vi "Measurement UI.vi"() -> ()   [LabVIEW 2025, in "Automotive Vision UI.lvlib"]
uses:
  Automotive Vision UI.lvlib
  <vilib>/gRPC/LabVIEW gRPC Library/Shared/grpcId.ctl
  <vilib>/vision/Image Controls.llb/IMAQ Image.ctl
  auto vision config.ctl
  Automotive-Vision-OOBService_client/RPC Messages/hwval_BoolRequest.ctl
  Automotive-Vision-OOBService_client/RPC Messages/hwval_ExportRequest.ctl
  Automotive-Vision-OOBService_client/RPC Messages/hwval_ExportTypeRequest.ctl
  Automotive-Vision-OOBService_client/RPC Messages/hwval_ExportFileType.ctl
  <vilib>/gRPC/LabVIEW gRPC Library/grpc-lvsupport-release.lvlib
  Automotive-Vision-OOBService_client/Automotive-Vision-OOBService_client.lvlib
panel:
  in  "REGISTERS":string[][](table)
  in  "FRAME COUNT BYTES":u32[](array[numeric]) format="%02x"
  in  "config":string
  out "WIDTH":u64
  out "HEIGHT":u64
  out "Numeric":i32
  out "error out":errorcluster
  in  "GRPC status":string
  out "OOB gRPC Port":i32
  in  "BITFILE":string="IMAGE RESOLUTION: 800x600 - RAW12"
  out "Available SI Devices":string[][](array[string])
  in  "RIO HANDLER":string
  out "BYTES ACQUIRED":u64 format="%#.6p"
  out "ERROR":bool
  out "IMAGE PIXEL DATA":u32[](array[numeric])
  in  "IMAGE SAVE FORMAT":u32(ring) items=["PNG", "RAW LLP"]
  out "FRAME COUNT":u64
  out "IMAGE DATA":string
  in  "PAUSE":bool
  in  "CAPTURE":bool
  in  "PATH TO IMAGE CAPTURE":path
  in  "SERIAL CHANNEL":string="SI1"
  out "SOURCE RATE (fps)":dbl
  out "STATE MESSAGE":string
  out "POC CURRENT (A)":dbl
  out "POC VOLTAGE (V)":dbl
  out "ACQ. DURATION (s)":dbl
  out "ACQ. IN PROGRESS":bool
  out "DISPLAY":T1(plugin-control)
  # "CONFIGURATION"
  # "Image path parameters"
  # "CONTROL"
  # "MONITOR"
  # "STATUS"
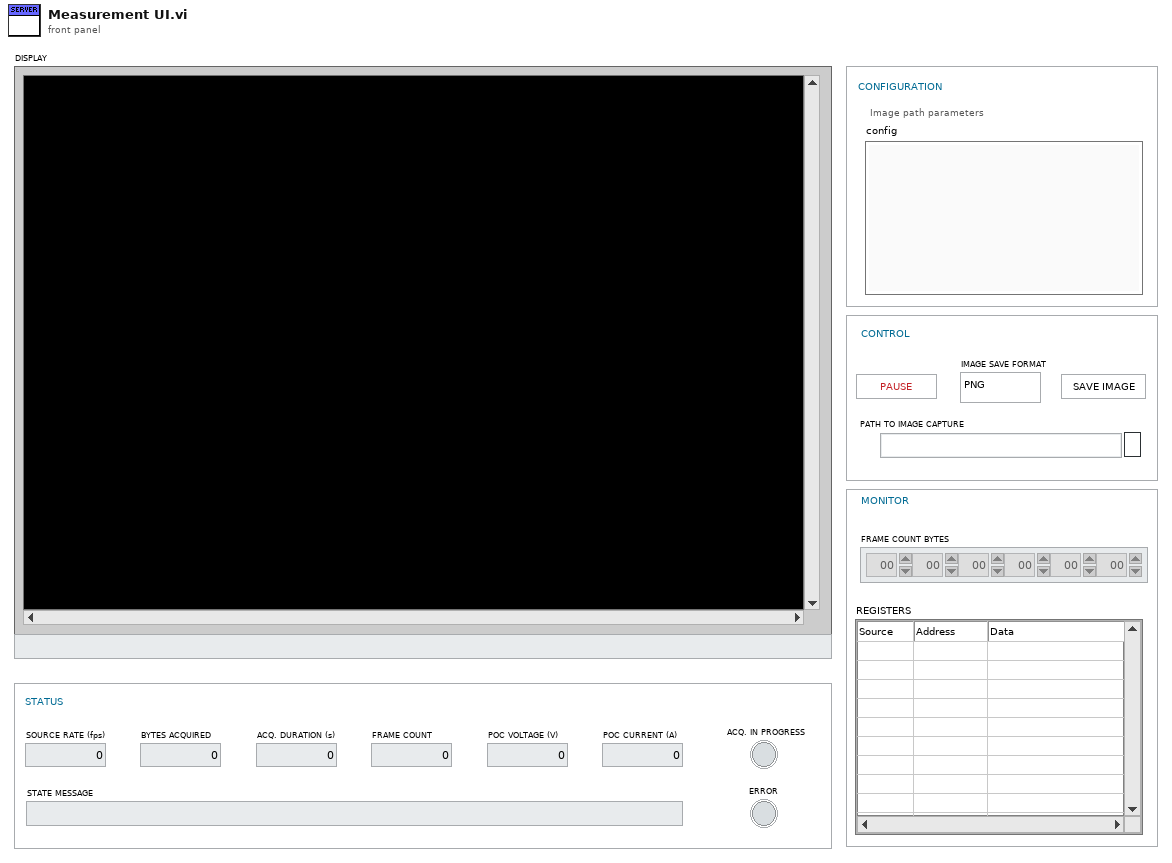
[diagram p1: front panel]
types:
  T1 = typedef "IMAQ Image.ctl" = refnum<image>
  T2 = typedef "Automotive Vision UI.lvlib/auto vision config.ctl" = cluster{"RIO Device":string, "Serial Channel":string, "SERDES Script":string, "POC Source":u32, "CSI-2 Data Source":u32, "Lane Count":u32, "Reference Clock":dbl, "Image Data Type":u32, "Interpretation":u32, "Pattern":u32, "Algorithm":u32, "Virtual Channel":u32, "Embedded Data":cluster{"Pre-embedded Lines":dbl, "Pre-embedded Line Length":dbl, "Post-embedded Lines":dbl, "Post-embedded Line Length":dbl, "Frame Count":cluster{"Line":dbl, "Offset":dbl, "Byte Count":dbl}}}
  T3 = typedef "grpc-lvsupport-release.lvlib/grpcId.ctl" = u64
  T4 = cluster{"pattern":i32, "algorithm":i32, "red gain":dbl, "green gain":dbl, "blue gain":dbl}
  T5 = typedef "Automotive-Vision-OOBService_client.lvlib/hwval_BoolRequest.ctl" = cluster{"BooleanData":bool}
  T6 = typedef "Automotive-Vision-OOBService_client.lvlib/hwval_ExportRequest.ctl" = cluster{"FilePath":string}
  T7 = typedef "Automotive-Vision-OOBService_client.lvlib/hwval_ExportTypeRequest.ctl" = cluster{"FileType":T8}
  T8 = typedef "Automotive-Vision-OOBService_client.lvlib/hwval_ExportFileType.ctl" = enum32{"EXPORT_PNG", "EXPORT_RAW"}
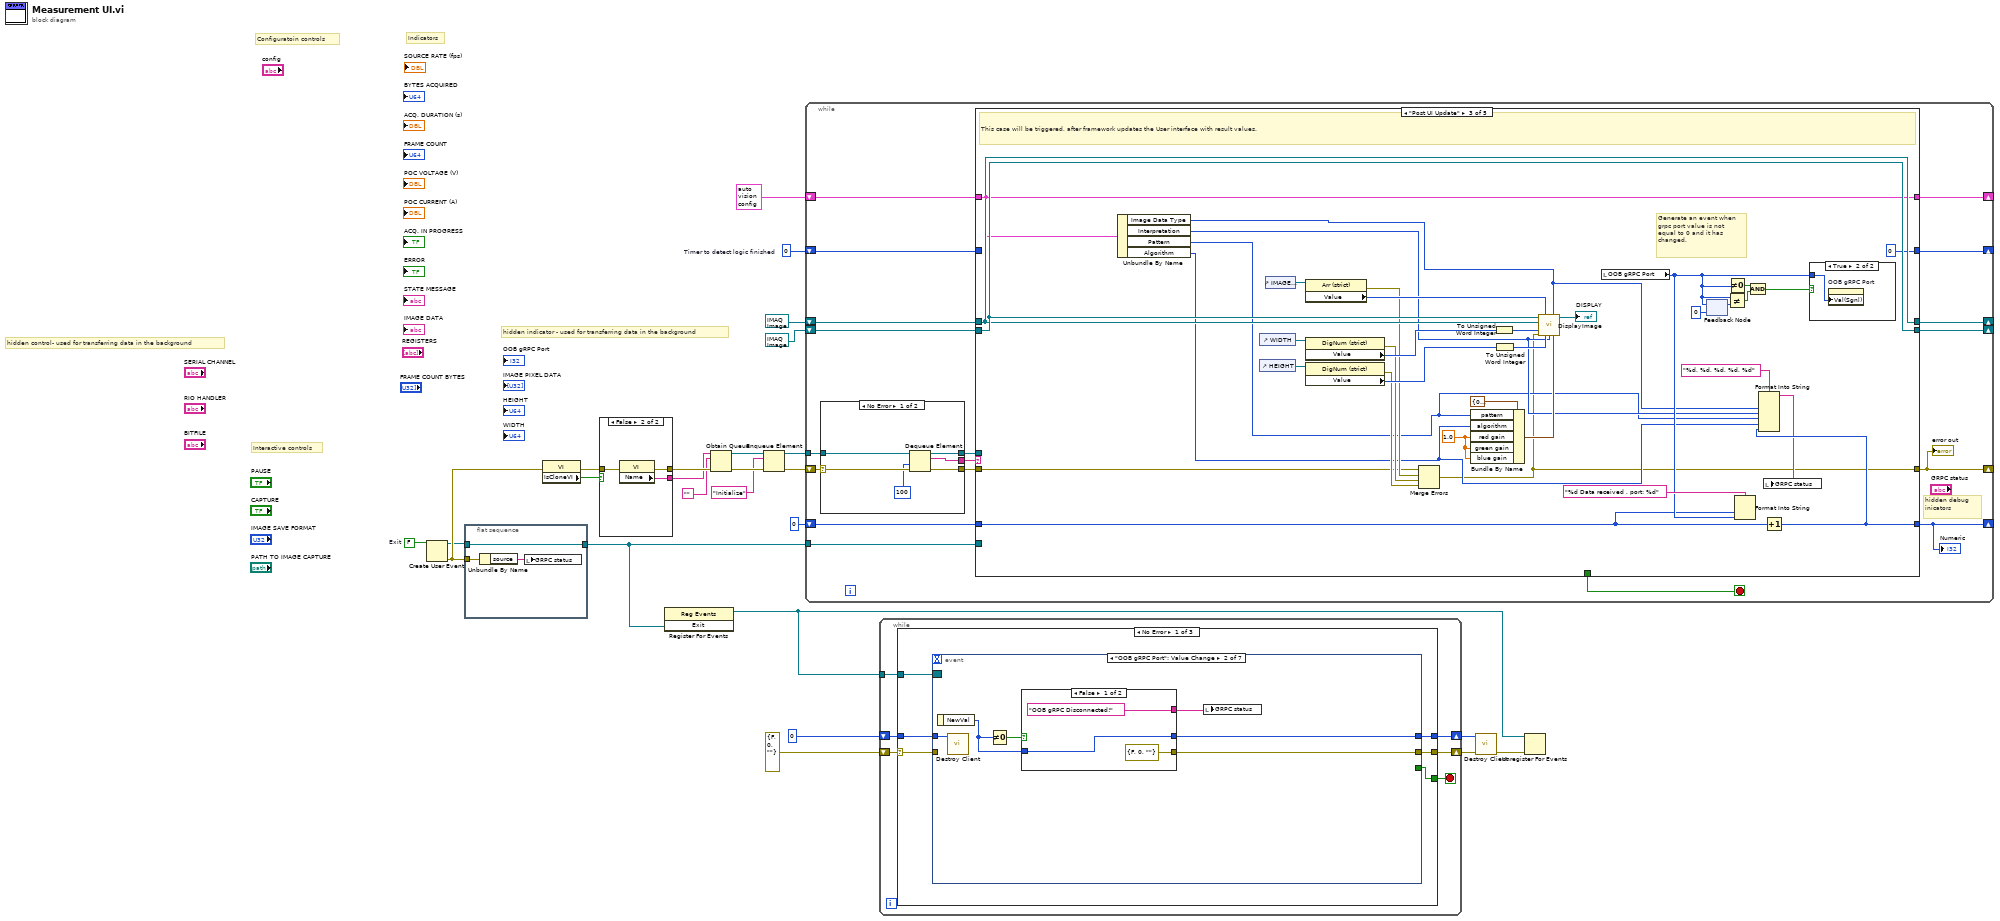
[diagram p0: block diagram]
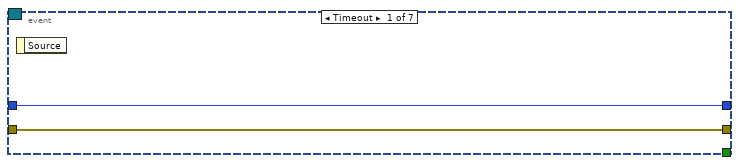
[diagram p2: hidden frame]
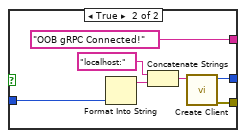
[diagram p3: hidden frame]
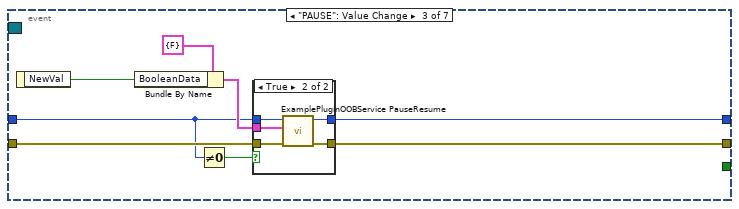
[diagram p4: hidden frame]
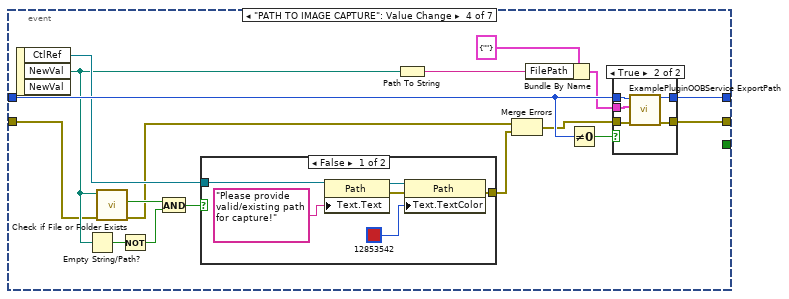
[diagram p6: hidden frame]
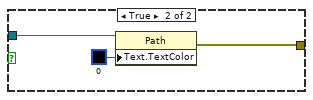
[diagram p7: hidden frame]
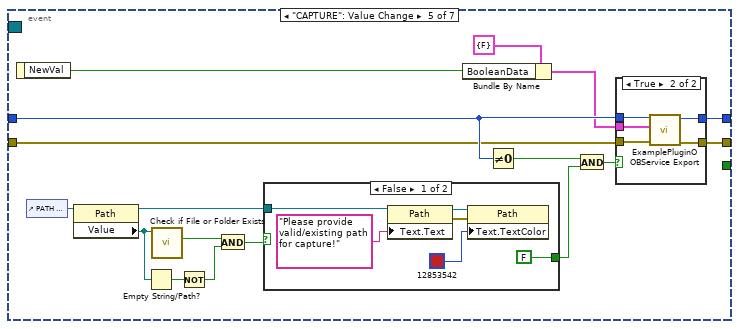
[diagram p9: hidden frame]
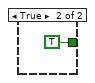
[diagram p10: hidden frame]
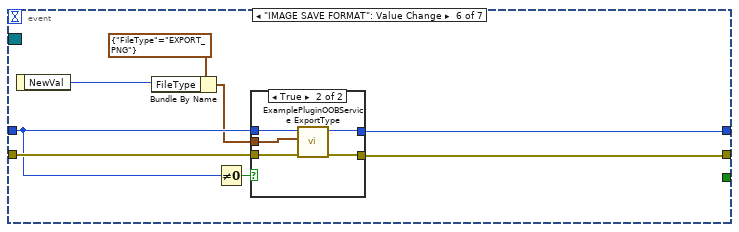
[diagram p12: hidden frame]
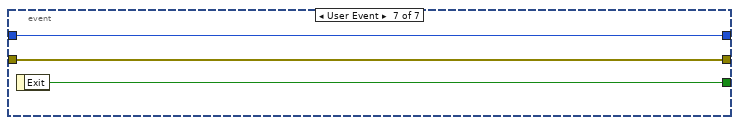
[diagram p14: hidden frame]
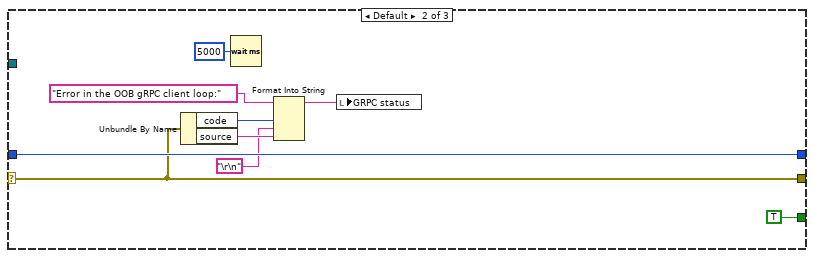
[diagram p15: hidden frame]
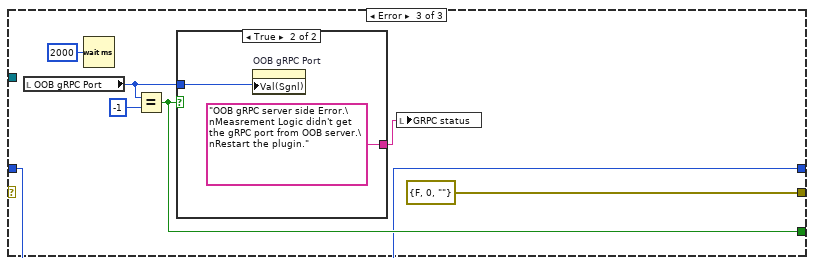
[diagram p16: hidden frame]
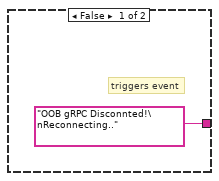
[diagram p17: hidden frame]
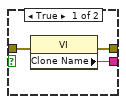
[diagram p18: hidden frame]
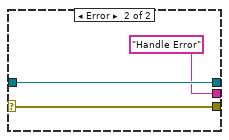
[diagram p19: hidden frame]
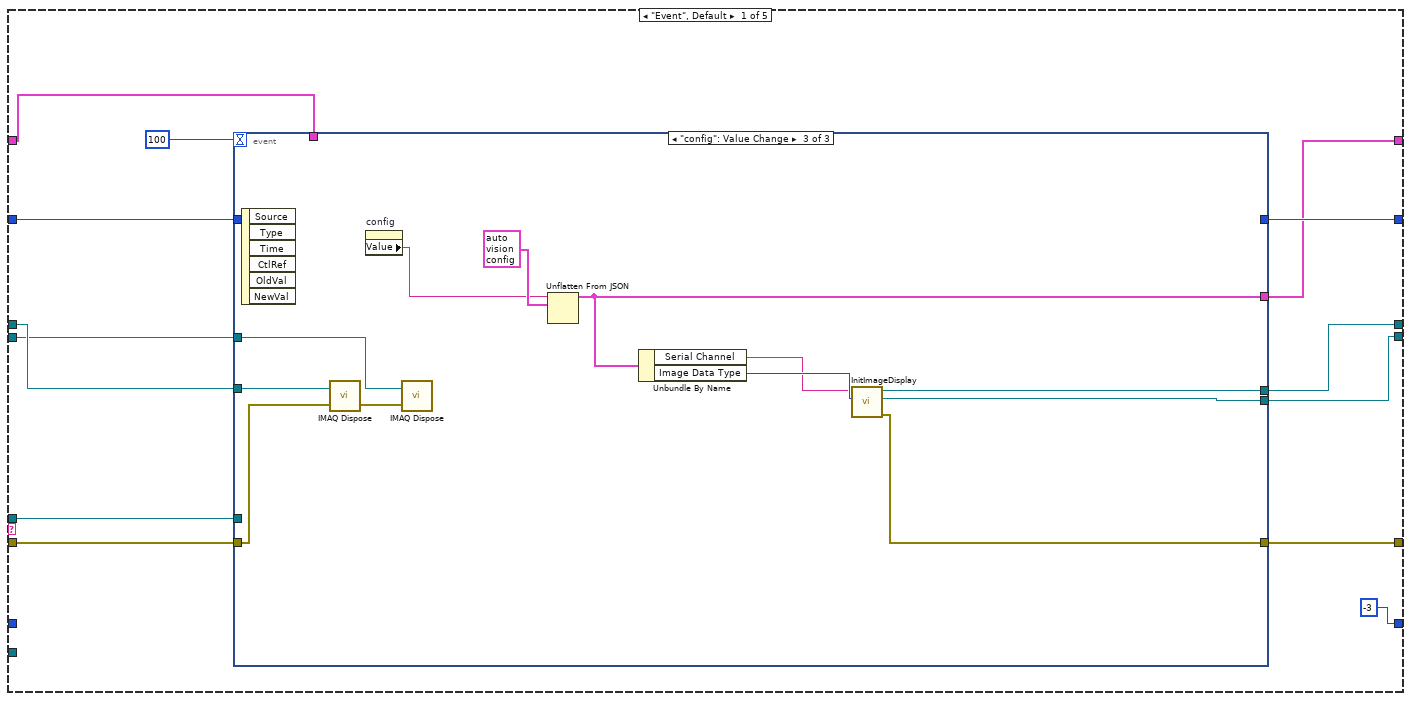
[diagram p20: hidden frame]
diagram:
  w6 = 0  # Timer to detect logic finished
  w15 = FALSE  # Exit
  # "Indicators"
  # "Configuratoin controls"
  # "Interactive controls"
  # "hidden indicator - used for transferring data in the background"
  # "hidden control- used for transferring data in the background"
  n1 = Create User Event(user event datatype=w15) -> (user event=w2:refnum<user-event>, error out=w8:errorcluster)  [unwired: 1 in]
  n2 = flat-sequence {
    tunnel: [w28] -> w9
    tunnel: w2 -> [w28]
    tunnel: w8 -> [w27]
    frame #0 {
      n3 = Unbundle By Name(w27) -> ("source"=w26:string)
      n4 = local write "GRPC status"(w26) -> ()
    }
  }
  n5 = property on="Property Node" class="VI"(error in=w8) -> (error out=w16:errorcluster, "IsCloneVI"=w17:bool)  [unwired: 1 in, 1 out]
  n6 = case shown="False" w17 {
    tunnel: [w31 w34] -> w25
    tunnel: [w30 w33] -> w24
    tunnel: w16 -> [w29 w32]
    frame True {
      n7 = property on="Property Node" class="VI"(error in=w29) -> (error out=w31:errorcluster, "Clone Name"=w30:string)  [unwired: 1 in, 1 out]
    }
    frame False {
      n8 = property on="Property Node" class="VI"(error in=w32) -> (error out=w34:errorcluster, "Name"=w33:string)  [unwired: 1 in, 1 out]
    }
  }
  n9 = register-events(w9) -> (reference out=w14:refnum<event-registration>)  [unwired: 2 in, 1 out]
  n10 = Obtain Queue(name (unnamed)=w24, element data type="" ("Empty String Constant"), error in (no error)=w25) -> (queue out=w21:refnum<queue>, error out=w23:errorcluster)  [unwired: 2 in, 1 out]
  n11 = Enqueue Element(queue=w21, element="Initialize", error in (no error)=w23) -> (queue out=w20:refnum<queue>, error out=w22:errorcluster)  [unwired: 1 in, 1 out]
  n12 = while {
    shift-right: [w41] -> _
    shift-left: w22 -> [w52]
    tunnel: w20 -> [w50]
    shift-right: [w43] -> _
    shift-left: T1 refnum ("Image Out Grayscale") -> [w45]
    shift-right: [w46] -> _
    shift-left: T1 refnum ("Image Out Grayscale") -> [w44]
    tunnel: w9 -> [w42]
    shift-right: [w39] -> _
    shift-left: 0 -> [w40]
    shift-right: [w37] -> _
    shift-left: w6 -> [w38]
    shift-right: [w35] -> _
    shift-left: T2 {"RIO Device"="", "Serial Channel"="", "SERDES Script"="", "POC Source"=0, "CSI-2 Data Source"=0, "Lane Count"=0, "Reference Clock"=0.0, "Image Data Type"=0, "Interpretation"=0, "Pattern"=0, "Algorithm"=0, "Virtual Channel"=0, "Embedded Data"={"Pre-embedded Lines"=0.0, "Pre-embedded Line Length"=0.0, "Post-embedded Lines"=0.0, "Post-embedded Line Length"=0.0, "Frame Count"={"Line"=0.0, "Offset"=0.0, "Byte Count"=0.0}}} ("Auto Vision Config") -> [w36]
    stop <- w47 stop-if-true
    # "hidden debug inicators"
    n13 = case shown="No Error" w52 {
      selector: w52 -> [w58 w61]
      tunnel: [w57 w61] -> w51
      tunnel: w50 -> [w56 w60]
      tunnel: [w55 w60] -> w49
      tunnel: [w54 "Handle Error"] -> w48
      frame No Error {
        n14 = Dequeue Element(queue=w56, timeout in ms (-1)=100, error in (no error)=w58) -> (queue out=w55:refnum<queue>, element=w54:string, error out=w57:errorcluster)  [unwired: 1 out]
      }
      frame Error {
      }
    }
    n15 = case shown="\"Post UI Update\"" w48 {
      tunnel: w51 -> [w73 w143 w172 w208 w247]
      tunnel: w49 -> [w71 _ _ w231 w246]
      tunnel: [w74 w140 w162 w202 w245] -> w41
      tunnel: [_ FALSE _ TRUE TRUE] -> w47
      tunnel: [w62 w139 w196 w224 w252] -> w46
      tunnel: [w63 w138 w194 w224 w253] -> w43
      tunnel: w45 -> [w65 _ w194 w225 w253]
      tunnel: w44 -> [w64 _ w196 w226 w252]
      tunnel: w42 -> [_ _ _ w212 _]
      tunnel: w40 -> [_ _ w182 _ _]
      tunnel: [-3 1 w164 -1 -2] -> w39
      tunnel: [w68 0 ("Numeric 2") 0 ("Numeric 2") 0 ("Numeric 2") 0 ("Numeric 2")] -> w37
      tunnel: w38 -> [w69 _ _ _ _]
      tunnel: w36 -> [w67 w132 w170 w199 w242]
      tunnel: [w66 w141 w170 w199 w242] -> w35
      frame "Event", Default {
        n16 = event shown="[2] \"config\": Value Change" {
          selector: _ -> [_ _ _]
          dyn-events: _ -> [_ _ _]
          timeout: 100 -> [_ _ _]
          tunnel: [w78 w117 w123] -> w74
          tunnel: w73 -> [w81 w118 w129]
          tunnel: w71 -> [w80 w116 _]
          tunnel: w69 -> [w87 _ _]
          tunnel: [w86 _ _] -> w68
          tunnel: w67 -> [w77 w114 _]
          tunnel: [w77 w114 w124] -> w66
          tunnel: w65 -> [w75 w112 w130]
          tunnel: w64 -> [w76 w113 w128]
          tunnel: [w75 w112 w126] -> w63
          tunnel: [w76 w113 w125] -> w62
          event Timeout {
            n17 = event-data() -> ()  [unwired: 1 in, 3 out]
            n18 = control-ref of="ACQ. IN PROGRESS"() -> (w83:refnum<vi>)
            n19 = Increment(x=w87) -> (x+1=w86:i32)
            n20 = property on="Property Node" class="Bool (strict)"(reference=w83) -> ("Value"=w82:bool)  [unwired: 1 in, 2 out]
            n21 = Greater?(x=w86, y=10) -> (0:w84:bool)
            n22 = And(x=w84, y=w82) -> (x .and. y?=w79:bool)
            n23 = case shown="True" w79 {
              tunnel: w81 -> [w88 w90]
              tunnel: w80 -> [_ _]
              tunnel: [w88 w92] -> w78
              frame False {
              }
              frame True {
                # "Only update status to done if no error happend"
                n24 = control-ref of="ACQ. IN PROGRESS"() -> (w93:refnum<vi>)
                n25 = property on="Property Node" class="Bool (strict)"(reference=w93, error in=w90, "Value"=FALSE) -> (error out=w89:errorcluster)  [unwired: 1 out]
                n26 = control-ref of="STATE MESSAGE"() -> (w94:refnum<vi>)
                n27 = property on="Property Node" class="Str"(reference=w94, error in=w89) -> (reference out=w102:refnum<vi>, error out=w96:errorcluster, "Value"=w101:string)
                n28 = Search and Replace String(case sensitive?=TRUE ("ignore case? (F)"), input string=w101, search string="error", error in=w96) -> (number of replacements=w98:i32, error out=w95:errorcluster)  [unwired: 4 in, 2 out]
                n29 = Equal To 0?(x=w98) -> (x = 0?=w97:bool)
                n30 = case shown="True" w97 {
                  tunnel: w102 -> [_ w109]
                  tunnel: w101 -> [_ w107]
                  tunnel: w95 -> [w103 w105]
                  tunnel: [w103 w106] -> w92
                  frame False {
                  }
                  frame True {
                    n31 = Search and Replace String(input string=w107, search string="^.*", replace string="Done" ("replace string (\"\")"), error in=w105) -> (result string=w108:string, error out=w104:errorcluster)  [unwired: 4 in, 2 out]
                    n32 = property on="Property Node" class="Str"(reference=w109, error in=w104, "Value"=w108) -> (error out=w106:errorcluster)  [unwired: 1 out]
                  }
                }
              }
            }
          }
          event Panel Close? {
            n33 = event-data() -> ()  [unwired: 1 in, 4 out]
            n34 = Enqueue Element(queue=w116, element="Exit", error in (no error)=w118) -> (error out=w117:errorcluster)  [unwired: 1 in, 2 out]
            n35 = event-data ("Event Filter Node")("Discard?"=TRUE) -> ()  [unwired: 1 in, 1 out]
          }
          event "config": Value Change {
            n36 = event-data() -> ()  [unwired: 1 in, 6 out]
            n37 = call "IMAQ Dispose"("Image"=w130, "error in (no error)"=w129) -> ("error out"=w127:errorcluster)  [unwired: 4 in]
            n38 = property on="config" class="Str"() -> ("Value"=w120:string)  [unwired: 2 in, 2 out]
            n39 = call "IMAQ Dispose"("Image"=w128, "error in (no error)"=w127) -> ()  [unwired: 4 in, 1 out]
            n40 = Unflatten From JSON(JSON string=w120, type and defaults=T2 {"RIO Device"="", "Serial Channel"="", "SERDES Script"="", "POC Source"=0, "CSI-2 Data Source"=0, "Lane Count"=0, "Reference Clock"=0.0, "Image Data Type"=0, "Interpretation"=0, "Pattern"=0, "Algorithm"=0, "Virtual Channel"=0, "Embedded Data"={"Pre-embedded Lines"=0.0, "Pre-embedded Line Length"=0.0, "Post-embedded Lines"=0.0, "Post-embedded Line Length"=0.0, "Frame Count"={"Line"=0.0, "Offset"=0.0, "Byte Count"=0.0}}} ("Auto Vision Config")) -> (value=w124:T2)  [unwired: 5 in, 1 out]
            n41 = Unbundle By Name(w124) -> ("Serial Channel"=w121:string, "Image Data Type"=w122:u32)
            n42 = call "InitImageDisplay.vi"("payload data type"=w122, "SI channel"=w121) -> ("error out"=w123:errorcluster, "Image Out Color"=w125:T1, "Image Out Grayscale"=w126:T1)  [unwired: 7 in]
          }
        }
      }
      frame "Initialize" {
        (unwired) 0
        # "Do a default selection for SI0"
        # "select SI cha."
        # "select 0. device in list"
        # "used to store device data between events"
        n43 = property on="config" class="Str"(error in=w143) -> (error out=w142:errorcluster, "Value"=w133:string)  [unwired: 1 in, 1 out]
        n44 = Empty String/Path?(string/path=w133) -> (empty?=w134:bool)
        n45 = case shown="False" w134 {
          tunnel: w133 -> [w159 _]
          tunnel: w142 -> [w158 _]
          tunnel: [w156 w160] -> w141
          tunnel: [w155 44] -> w136
          tunnel: w132 -> [_ w160]
          frame False {
            n46 = Unflatten From JSON(JSON string=w159, type and defaults=T2 {"RIO Device"="", "Serial Channel"="", "SERDES Script"="", "POC Source"=0, "CSI-2 Data Source"=0, "Lane Count"=0, "Reference Clock"=0.0, "Image Data Type"=0, "Interpretation"=0, "Pattern"=0, "Algorithm"=0, "Virtual Channel"=0, "Embedded Data"={"Pre-embedded Lines"=0.0, "Pre-embedded Line Length"=0.0, "Post-embedded Lines"=0.0, "Post-embedded Line Length"=0.0, "Frame Count"={"Line"=0.0, "Offset"=0.0, "Byte Count"=0.0}}} ("Auto Vision Config"), error in (no error)=w158) -> (value=w156:T2)  [unwired: 4 in, 1 out]
            n47 = Unbundle By Name(w156) -> ("Image Data Type"=w155:u32)
          }
          frame True {
          }
        }
        n48 = call "GetChimeraResources.vi"("error in (no error)"=w143) -> ("error out"=w137:errorcluster, "Available input channels on Automotive Camera Vision Devices"=w152:string[][])  [unwired: 7 in, 2 out]
        "Available SI Devices" <- w152
        n49 = Index Array(array=w152) -> (element=w148:string[])  [unwired: 2 in]
        n50 = Array Subset(array=w148, index=2) -> (w151:string[])  [unwired: 1 in]
        n51 = Index Array(array=w148, index #1=0 ("index"), index #2=1 ("index")) -> (element #1=w149:string, element #2=w145:string)
        n52 = Index Array(array=w151) -> (element=w135:string)  [unwired: 1 in]
        n53 = local write "RIO HANDLER"(w149) -> ()
        n54 = local write "BITFILE"(w145) -> ()
        n55 = local write "SERIAL CHANNEL"(w135) -> ()
        n56 = call "InitImageDisplay.vi"("error in (no error)"=w137, "payload data type"=w136, "SI channel"=w135) -> ("error out"=w140:errorcluster, "Image Out Color"=w139:T1, "Image Out Grayscale"=w138:T1)  [unwired: 6 in]
      }
      frame "Post UI Update" {
        w191 = 1.0 ("red gain")
        # "Generate an event when grpc port value is not equal to 0 and it has changed."
        # "This case will be triggered, after framework updates the User interface with result values."
        n57 = Unbundle By Name(w170) -> ("Image Data Type"=w168:u32, "Interpretation"=w167:u32, "Pattern"=w166:u32, "Algorithm"=w165:u32)
        n58 = control-ref of="WIDTH"() -> (w181:refnum<vi>)
        n59 = control-ref of="HEIGHT"() -> (w180:refnum<vi>)
        n60 = control-ref of="IMAGE PIXEL DATA"() -> (w197:refnum<vi>)
        n61 = property on="Property Node" class="Arr (strict)"(reference=w197) -> (error out=w175:errorcluster, "Value"=w193:u32[])  [unwired: 1 in, 1 out]
        n62 = property on="Property Node" class="DigNum (strict)"(reference=w181) -> (error out=w174:errorcluster, "Value"=w179:u64)  [unwired: 1 in, 1 out]
        n63 = property on="Property Node" class="DigNum (strict)"(reference=w180) -> (error out=w173:errorcluster, "Value"=w177:u64)  [unwired: 1 in, 1 out]
        n64 = Merge Errors(w172, w175, w174, w173) -> (w162:errorcluster)
        n65 = Bundle By Name(cluster=T4 {"pattern"=0, "algorithm"=0, "red gain"=0.0, "green gain"=0.0, "blue gain"=0.0} ("bayer parameters"), "pattern"=w166, "algorithm"=w165, "red gain"=w191, "green gain"=w191, "blue gain"=w191) -> (w190:T4)
        n66 = To Unsigned Word Integer(number=w179) -> (unsigned 16bit integer=w178:u16)
        n67 = To Unsigned Word Integer(number=w177) -> (unsigned 16bit integer=w176:u16)
        n68 = call "DisplayImage.vi"("image color"=w196, "Image Pixel Data"=w193, "data type"=w168, "Image grayscale"=w194, "width"=w178, "error in (no error)"=w162, "height"=w176, "interpretation"=w167, "bayer parameters"=w190) -> ("display image"=→"DISPLAY":T1)  [unwired: 5 in, 1 out]
        n69 = local read "OOB gRPC Port"() -> (w183:i32)
        n70 = feedback #1(0 ("OOB gRPC Port")) -> (w186:i32)
        n71 = feedback-in #1(w183) -> ()
        n72 = Not Equal?(x=w183, y=w186) -> (x != y?=w187:bool)
        n73 = Not Equal To 0?(x=w183) -> (x != 0?=w188:bool)
        n74 = Format Into String(format string="%d Data received , port: %d" ("GRPC status"), w182, w183) -> ()  [unwired: 2 in, 2 out]
        n75 = Compound Arithmetic op=AND(w188, w187) -> (w185:bool)
        n76 = Increment(x=w182) -> (x+1=w164:i32)
        n77 = Format Into String(format string="%d, %d, %d, %d, %d" ("GRPC status"), w168, w167, w166, w165, w164) -> (resulting string=w163:string)  [unwired: 2 in, 1 out]
        n78 = local write "GRPC status"(w163) -> ()
        n79 = case shown="True" w185 {
          tunnel: w183 -> [_ w198]
          frame False {
          }
          frame True {
            n80 = property on="OOB gRPC Port" class="DigNum (strict)"("Val(Sgnl)"=w198) -> ()  [unwired: 2 in, 2 out]
          }
        }
      }
      frame "Exit" {
        w224 = T1 refnum ("Image Out Grayscale")
        # "Only update status to done if no error happend"
        # "This case is triggered to close the User Interface from framework"
        n81 = call "IMAQ Dispose"("Image"=w226) -> ("error out"=w227:errorcluster)  [unwired: 5 in]
        n82 = Flush Queue(queue=w231, error in (no error)=w208) -> (queue out=w230:refnum<queue>, error out=w229:errorcluster)  [unwired: 1 out]
        n83 = Generate User Event(user event=w212, event data cluster=TRUE ("event data")) -> (user event out=w213:refnum<user-event>, error out=w200:errorcluster)  [unwired: 2 in]
        n84 = call "IMAQ Dispose"("Image"=w225, "error in (no error)"=w227) -> ("error out"=w207:errorcluster)  [unwired: 4 in]
        n85 = Release Queue(queue=w230, force destroy? (F)=TRUE, error in (no error)=w229) -> (error out=w211:errorcluster)  [unwired: 2 out]
        n86 = Destroy User Event(user event=w213, error in=w200) -> (error out=w210:errorcluster)
        n87 = Merge Errors(w207, w211, w210) -> (w206:errorcluster)
        n88 = control-ref of="ACQ. IN PROGRESS"() -> (w223:refnum<vi>)
        n89 = property on="Property Node" class="Bool (strict)"(reference=w223, error in=w206, "Value"=FALSE) -> (error out=w205:errorcluster)  [unwired: 1 out]
        n90 = control-ref of="STATE MESSAGE"() -> (w221:refnum<vi>)
        n91 = property on="Property Node" class="Str"(reference=w221, error in=w205) -> (reference out=w220:refnum<vi>, error out=w204:errorcluster, "Value"=w219:string)
        n92 = Search and Replace String(case sensitive?=TRUE ("ignore case? (F)"), input string=w219, search string="error", error in=w204) -> (number of replacements=w216:i32, error out=w203:errorcluster)  [unwired: 4 in, 2 out]
        n93 = Equal To 0?(x=w216) -> (x = 0?=w215:bool)
        n94 = case shown="False" w215 {
          tunnel: w220 -> [_ w239]
          tunnel: w219 -> [_ w237]
          tunnel: w203 -> [w233 w235]
          tunnel: [w233 w236] -> w202
          frame False {
          }
          frame True {
            n95 = Search and Replace String(input string=w237, search string="^.*", replace string="Done" ("replace string (\"\")"), error in=w235) -> (result string=w238:string, error out=w234:errorcluster)  [unwired: 4 in, 2 out]
            n96 = property on="Property Node" class="Str"(reference=w239, error in=w234, "Value"=w238) -> (error out=w236:errorcluster)  [unwired: 1 out]
          }
        }
      }
      frame "Handle Error" {
        n97 = Flush Queue(queue=w246, error in (no error)=w247) -> (queue out=w250:refnum<queue>, error out=w249:errorcluster)  [unwired: 1 out]
        n98 = Release Queue(queue=w250, force destroy? (F)=TRUE, error in (no error)=w249) -> (error out=w245:errorcluster)  [unwired: 2 out]
      }
    }
    "error out" <- w41
    "Numeric" <- w39
  }
  n99 = while {
    tunnel: w14 -> [w256]
    shift-right: [w257] -> w12
    shift-left: errorcluster {"status"=FALSE, "code"=0, "source"=""} ("error IO") -> [w259]
    shift-right: [w254] -> w10
    shift-left: T3 0 ("gRPC ID out") -> [w255]
    stop <- w258 stop-if-true
    n100 = case shown="No Error" w259 {
      selector: w259 -> [w263 w383 _]
      tunnel: [w260 TRUE w395] -> w258
      tunnel: [w264 w383 errorcluster {"status"=FALSE, "code"=0, "source"=""} ("error IO")] -> w257
      tunnel: w256 -> [w265 _ _]
      tunnel: w255 -> [w262 w388 w393]
      tunnel: [w261 w388 w393] -> w254
      frame No Error {
        n101 = event shown="[1] \"OOB gRPC Port\": Value Change" {
          selector: w265 -> [_ _ _ _ _ _ _]
          dyn-events: _ -> [_ _ _ _ _ _ _]
          timeout: _ -> [_ _ _ _ _ _ _]
          tunnel: [w267 w273 w290 w314 w348 w368 w378] -> w264
          tunnel: w263 -> [w267 _ w289 w299 w341 w369 w378]
          tunnel: w262 -> [w266 w269 w285 w312 w347 w367 w379]
          tunnel: [w266 w272 w291 w315 w346 w366 w379] -> w261
          tunnel: [_ _ _ _ _ _ w380] -> w260
          event Timeout {
            n102 = event-data() -> ()  [unwired: 1 in, 1 out]
          }
          event "OOB gRPC Port": Value Change {
            n103 = event-data() -> ("NewVal"=w270:i32)  [unwired: 1 in]
            n104 = call "Destroy Client.vi"("gRPC ID"=w269) -> ()  [unwired: 10 in, 1 out]
            n105 = Not Equal To 0?(x=w270) -> (x != 0?=w271:bool)
            n106 = case shown="False" w271 {
              tunnel: [errorcluster {"status"=FALSE, "code"=0, "source"=""} ("error out") w277] -> w273
              tunnel: w270 -> [w276 w281]
              tunnel: [w276 w278] -> w272
              tunnel: ["OOB gRPC Disconnected!" ("Status") "OOB gRPC Connected!" ("Status")] -> w268
              frame False {
              }
              frame True {
                n107 = Format Into String(w281) -> (resulting string=w283:string)  [unwired: 3 in, 1 out]
                n108 = Concatenate Strings("localhost:" ("string"), w283) -> (w279:string)
                n109 = call "Create Client.vi"("address"=w279) -> ("error out"=w277:errorcluster, "gRPC ID Out"=w278:T3)  [unwired: 9 in]
              }
            }
            n110 = local write "GRPC status"(w268) -> ()
          }
          event "PAUSE": Value Change {
            n111 = event-data() -> ("NewVal"=w287:bool)  [unwired: 1 in]
            n112 = Bundle By Name(cluster=T5 {"BooleanData"=FALSE} ("Request Data"), "BooleanData"=w287) -> (w288:T5)
            n113 = Not Equal To 0?(x=w285) -> (x != 0?=w286:bool)
            n114 = case shown="True" w286 {
              tunnel: [w293 w297] -> w291
              tunnel: [w292 w296] -> w290
              tunnel: w285 -> [w293 w298]
              tunnel: w289 -> [w292 w295]
              tunnel: w288 -> [_ w294]
              frame False {
              }
              frame True {
                n115 = call "ExamplePluginOOBService PauseResume.vi"("error in"=w295, "Request Data"=w294, "gRPC ID"=w298) -> ("error out"=w296:errorcluster, "gRPC ID out"=w297:T3)  [unwired: 6 in, 1 out]
              }
            }
          }
          event "PATH TO IMAGE CAPTURE": Value Change {
            n116 = event-data() -> ("CtlRef"=w308:refnum<vi>, "NewVal"=w304:path)  [unwired: 1 in, 1 out]
            n117 = Empty String/Path?(string/path=w304) -> (empty?=w307:bool)
            n118 = call <vilib>:"Check if File or Folder Exists.vi"("error in (no error)"=w299, "path"=w304) -> ("error out"=w300:errorcluster, "file or folder exists?"=w306:bool)  [unwired: 7 in, 1 out]
            n119 = Not(x=w307) -> (.not. x?=w305:bool)
            n120 = And(x=w306, y=w305) -> (x .and. y?=w303:bool)
            n121 = case shown="False" w303 {
              tunnel: w308 -> [w321 w324]
              tunnel: [w316 w322] -> w301
              frame False {
                n122 = property on="Property Node" class="Path"(reference=w321, "Text.Text"="Please provide valid/existing path for capture!" ("Path Text.Text")) -> (reference out=w320:refnum<vi>, error out=w319:errorcluster)  [unwired: 1 in]
                n123 = property on="Property Node" class="Path"(reference=w320, error in=w319, "Text.TextColor"=u32 12853542 ("Path Text.Text Colors:Text Color")) -> (error out=w316:errorcluster)  [unwired: 1 out]
              }
              frame True {
                n124 = property on="Property Node" class="Path"(reference=w324, "Text.TextColor"=u32 0 ("Path Text.Text Colors:Text Color")) -> (error out=w322:errorcluster)  [unwired: 1 in, 1 out]
              }
            }
            n125 = Path To String(path=w304) -> (string=w310:string)
            n126 = Merge Errors(w300, w301) -> (w302:errorcluster)
            n127 = Bundle By Name(cluster=T6 {"FilePath"=""} ("Request Data"), "FilePath"=w310) -> (w309:T6)
            n128 = Not Equal To 0?(x=w312) -> (x != 0?=w313:bool)
            n129 = case shown="True" w313 {
              tunnel: [w326 w330] -> w315
              tunnel: [w325 w328] -> w314
              tunnel: w312 -> [w326 w331]
              tunnel: w302 -> [w325 w329]
              tunnel: w309 -> [_ w327]
              frame False {
              }
              frame True {
                n130 = call "ExamplePluginOOBService ExportPath.vi"("error in"=w329, "Request Data"=w327, "gRPC ID"=w331) -> ("error out"=w328:errorcluster, "gRPC ID out"=w330:T3)  [unwired: 6 in, 1 out]
              }
            }
          }
          event "CAPTURE": Value Change {
            n131 = event-data() -> ("NewVal"=w344:bool)  [unwired: 1 in]
            n132 = control-ref of="PATH TO IMAGE CAPTURE"() -> (w337:refnum<vi>)
            n133 = property on="Property Node" class="Path"(reference=w337) -> (reference out=w342:refnum<vi>, "Value"=w336:path)  [unwired: 1 in, 1 out]
            n134 = Empty String/Path?(string/path=w336) -> (empty?=w335:bool)
            n135 = call <vilib>:"Check if File or Folder Exists.vi"("path"=w336) -> ("file or folder exists?"=w333:bool)  [unwired: 8 in, 2 out]
            n136 = Not(x=w335) -> (.not. x?=w332:bool)
            n137 = And(x=w333, y=w332) -> (x .and. y?=w334:bool)
            n138 = case shown="False" w334 {
              tunnel: w342 -> [w354 _]
              tunnel: [FALSE TRUE] -> w338
              frame False {
                n139 = property on="Property Node" class="Path"(reference=w354, "Text.Text"="Please provide valid/existing path for capture!" ("Path Text.Text")) -> (reference out=w353:refnum<vi>, error out=w352:errorcluster)  [unwired: 1 in]
                n140 = property on="Property Node" class="Path"(reference=w353, error in=w352, "Text.TextColor"=u32 12853542 ("Path Text.Text Colors:Text Color")) -> ()  [unwired: 2 out]
              }
              frame True {
              }
            }
            n141 = Bundle By Name(cluster=T5 {"BooleanData"=FALSE} ("Request Data"), "BooleanData"=w344) -> (w343:T5)
            n142 = Not Equal To 0?(x=w347) -> (x != 0?=w340:bool)
            n143 = And(x=w340, y=w338) -> (x .and. y?=w339:bool)
            n144 = case shown="True" w339 {
              tunnel: w341 -> [w356 w362]
              tunnel: [w356 w361] -> w348
              tunnel: w347 -> [w357 w360]
              tunnel: [w357 w359] -> w346
              tunnel: w343 -> [_ w358]
              frame False {
              }
              frame True {
                n145 = call "ExamplePluginOOBService Export.vi"("error in"=w362, "Request Data"=w358, "gRPC ID"=w360) -> ("error out"=w361:errorcluster, "gRPC ID out"=w359:T3)  [unwired: 6 in, 1 out]
              }
            }
          }
          event "IMAGE SAVE FORMAT": Value Change {
            n146 = event-data() -> ("NewVal"=w364:u32)  [unwired: 1 in]
            n147 = Bundle By Name(cluster=T7 {"FileType"=enum."EXPORT_PNG"} ("Request Data"), "FileType"=w364) -> (w363:T7)
            n148 = Not Equal To 0?(x=w367) -> (x != 0?=w370:bool)
            n149 = case shown="True" w370 {
              tunnel: w369 -> [w371 w375]
              tunnel: [w371 w374] -> w368
              tunnel: w367 -> [w372 w376]
              tunnel: [w372 w373] -> w366
              tunnel: w363 -> [_ w377]
              frame False {
              }
              frame True {
                n150 = call "ExamplePluginOOBService ExportType.vi"("error in"=w375, "Request Data"=w377, "gRPC ID"=w376) -> ("error out"=w374:errorcluster, "gRPC ID out"=w373:T3)  [unwired: 6 in, 1 out]
              }
            }
          }
          event User Event {
            n151 = event-data() -> ("Exit"=w380:bool)  [unwired: 1 in]
          }
        }
      }
      frame Default {
        n152 = Unbundle By Name(w383) -> ("code"=w387:i32, "source"=w386:string)
        n153 = Wait (ms)(milliseconds to wait=u32 5000) -> ()  [unwired: 1 out]
        n154 = Format Into String(initial string="Error in the OOB gRPC client loop:" ("format string"), w387, "\r\n" ("End of Line Constant"), w386) -> (resulting string=w381:string)  [unwired: 2 in, 1 out]
        n155 = local write "GRPC status"(w381) -> ()
      }
      frame Error {
        n156 = local read "OOB gRPC Port"() -> (w391:i32)
        n157 = Wait (ms)(milliseconds to wait=u32 2000) -> ()  [unwired: 1 out]
        n158 = Equal?(x=w391, y=-1 ("x")) -> (x = y?=w395:bool)
        n159 = case shown="True" w395 {
          tunnel: ["OOB gRPC Disconnted!\nReconnecting.." ("Status") "OOB gRPC server side Error.\nMeasrement Logic didn't get the gRPC port from OOB server.\nRestart the plugin." ("Status")] -> w390
          tunnel: w391 -> [_ w398]
          frame False {
            # "triggers event"
          }
          frame True {
            n160 = property on="OOB gRPC Port" class="DigNum (strict)"("Val(Sgnl)"=w398) -> ()  [unwired: 2 in, 2 out]
          }
        }
        n161 = local write "GRPC status"(w390) -> ()
      }
    }
  }
  n162 = call "Destroy Client.vi"("error in"=w12, "gRPC ID"=w10) -> ("error out"=w11:errorcluster)  [unwired: 9 in]
  n163 = Unregister For Events(event registration refnum=w14, error in=w11) -> ()  [unwired: 1 out]
